vi "Kinesis-Teste-Vector-1.vi"() -> ()   [LabVIEW 2014]
doc: "André Romero - 2017\nandretec@ifsc.usp.br"
uses:
  C:/users-lab/Andre/GITs/andretec/Thorlabs-Vector-Move/kinesisTec/Kinesis/Thorlabs.MotionControl.Controls.dll
  Kinesis/Thorlabs.MotionControl.Controls.dll
  C:/users-lab/Andre/GITs/andretec/Thorlabs-Vector-Move/kinesisTec/Kinesis/Thorlabs.MotionControl.TCube.DCServoCLI.dll
  Kinesis/Thorlabs.MotionControl.TCube.DCServoCLI.dll
  C:/users-lab/Andre/GITs/andretec/Thorlabs-Vector-Move/kinesisTec/Kinesis/Thorlabs.MotionControl.GenericMotorCLI.dll
  Kinesis/Thorlabs.MotionControl.GenericMotorCLI.dll
  Basic-VIs/motorsGlobalVar.vi
  <vilib>/Instr/_visa.llb/VISA Configure Serial Port (Instr).vi
panel:
  out "IsAtHWLimit":bool
  out "CanMoveContinuous":bool
  out "GetLimitsSoftwareApproachPolicy":i16(ring) items=["DisallowIllegalMoves", "AllowPartialMoves", "AllowAllMoves"]
  in  "stop":bool
  in  "Adjust Motors":bool
  out "Process time":string="0:00:50"
  out "Progress %":dbl(slide) scale=0.0..100.0
  out "XY Graph":cluster{"Graph X":dbl[], "Graph Y":dbl[]}(graph)
  in  "Swap XY":bool
  out "stop cronometro":bool=TRUE
  in  "Stop Button":bool
  in  "Graph Y":dbl[](array[numeric])=[0.0, 0.0, 6.6674440298507465, 6.6674440298507465, 6.6674440298507465, 6.6674440298507465, 6.6674440298507465, 6.6674440298507465, 6.6674440298507465, 6.6674440298507465, 6.6674440298507465, 6.6674440298507465, 6.6674440298507465, 6.6674440298507465, 6.6674440298507465, 6.6674440298507465, 6.6674440298507465, 6.6674440298507465, 6.6674440298507465, 6.6674440298507465, 6.6674440298507465, 6.6674440298507465, 6.6674440298507465, 6.6674440298507465, 6.6674440298507465, 6.6674440298507465, 6.6674440298507465, 6.6674440298507465, 6.6674440298507465, 6.6674440298507465, 6.6674440298507465, 6.6674440298507465, 6.6674440298507465, 6.6674440298507465, 6.6674440298507465, 6.6674440298507465, 6.6674440298507465, 6.6674440298507465, 6.6674440298507465, 6.6674440298507465, 6.6674440298507465, 6.6674440298507465, 6.6674440298507465, 6.673128498134329, 6.673128498134329, 6.673128498134329, 6.673128498134329, 6.673128498134329, 6.687354244402985, 6.687354244402985, 6.687354244402985, 6.687354244402985, 6.687354244402985, 6.692543143656716, 6.692543143656716, 6.692543143656716, 6.692543143656716, 6.692543143656716, 6.692543143656716, 6.692543143656716, 6.692543143656716, 6.692543143656716, 6.692543143656716, 6.692543143656716, 6.692543143656716, 6.691522854477612, 6.691522854477612, 6.691522854477612, 6.691522854477612, 6.691522854477612, 6.680183069029851, 6.680183069029851, 6.680183069029851, 6.680183069029851, 6.680183069029851, 6.658640391791045, 6.658640391791045, 6.658640391791045, 6.658640391791045, 6.658640391791045, 6.644793610074627, 6.644793610074627, 6.644793610074627, 6.644793610074627, 6.644793610074627, 6.642490671641791, 6.642490671641791, 6.642490671641791, 6.642490671641791, 6.642490671641791, 6.642490671641791, 6.642490671641791, 6.642490671641791, 6.642490671641791, 6.642490671641791, 6.642490671641791, 6.642490671641791, 6.642490671641791, 6.642490671641791, 6.642490671641791, 6.647825326492537, 6.647825326492537, 6.647825326492537, 6.647825326492537, 6.647825326492537, 6.66543260261194, 6.66543260261194, 6.66543260261194, 6.66543260261194, 6.66543260261194, 6.685226212686567, 6.685226212686567, 6.685226212686567, 6.685226212686567, 6.685226212686567, 6.692484841417911, 6.692484841417911, 6.692484841417911, 6.692484841417911, 6.692484841417911, 6.692543143656716, 6.692543143656716, 6.692543143656716, 6.692543143656716, 6.692543143656716, 6.692543143656716, 6.692543143656716, 6.691464552238806, 6.691464552238806, 6.691464552238806, 6.691464552238806, 6.691464552238806, 6.679833255597015, 6.679833255597015, 6.679833255597015, 6.679833255597015, 6.679833255597015, 6.658057369402985, 6.658057369402985, 6.658057369402985, 6.658057369402985, 6.658057369402985, 6.644647854477612, 6.644647854477612, 6.644647854477612, 6.644647854477612, 6.644647854477612, 6.642548973880597, 6.642548973880597, 6.642548973880597, 6.642548973880597, 6.642548973880597, 6.642519822761194, 6.642519822761194, 6.642519822761194, 6.642519822761194, 6.642519822761194, 6.642519822761194, 6.642519822761194, 6.642519822761194, 6.643569263059701, 6.643569263059701, 6.643569263059701, 6.643569263059701, 6.643569263059701, 6.655521222014926, 6.655521222014926, 6.655521222014926, 6.655521222014926, 6.655521222014926, 6.677180503731344, 6.677180503731344, 6.677180503731344, 6.677180503731344, 6.677180503731344, 6.690531716417911, 6.690531716417911, 6.690531716417911, 6.690531716417911, 6.690531716417911, 6.692572294776119, 6.692572294776119, 6.692572294776119, 6.692572294776119, 6.692572294776119, 6.692572294776119, 6.692572294776119, 6.692572294776119, 6.692572294776119, 6.692572294776119, 6.692572294776119, 6.692572294776119, 6.691522854477612, 6.691522854477612, 6.691522854477612, 6.691522854477612, 6.691522854477612, 6.680008162313433, 6.680008162313433, 6.680008162313433, 6.680008162313433, 6.680008162313433, 6.668668376865671, 6.668668376865671, 6.668668376865671, 6.668668376865671, 6.668668376865671, 6.667502332089552, 6.667502332089552, 6.667502332089552, 6.667502332089552, 6.667502332089552, 6.667502332089552, 6.667502332089552, 6.667502332089552, 6.667502332089552, 6.667502332089552, 6.667502332089552, 6.667502332089552, 6.667531483208955, 6.667531483208955, 6.667531483208955, 6.667531483208955, 6.667531483208955, 6.667531483208955, 6.667531483208955, 6.667531483208955, 6.667531483208955, 6.667531483208955, 6.667531483208955, 6.667531483208955, 6.667531483208955, 6.667531483208955, 6.667531483208955, 6.667531483208955, 6.667531483208955, 6.667531483208955, 6.667531483208955, 6.667531483208955, 6.667531483208955, 6.667531483208955, 6.667531483208955, 6.667531483208955, 6.667531483208955, 6.667531483208955, 6.667531483208955, 6.667531483208955, 6.667531483208955, 6.667531483208955, 6.667531483208955, 6.667531483208955, 6.667531483208955, 6.667531483208955, 6.667531483208955, 6.667531483208955, 6.667531483208955, 6.6663945895522385, 6.6663945895522385, 6.6663945895522385, 6.6663945895522385, 6.6663945895522385, 6.662051072761194, 6.662051072761194, 6.662051072761194, 6.662051072761194, 6.662051072761194, 6.644035680970149, 6.644035680970149, 6.644035680970149, 6.644035680970149, 6.644035680970149, 6.606430736940299, 6.606430736940299, 6.606430736940299, 6.606430736940299, 6.606430736940299, 6.593924906716418, 6.593924906716418, 6.593924906716418, 6.593924906716418, 6.593924906716418, 6.574539412313433, 6.574539412313433, 6.574539412313433, 6.574539412313433, 6.574539412313433, 6.567484841417911, 6.567484841417911, 6.567484841417911, 6.567484841417911, 6.567484841417911, 6.567484841417911, 6.567484841417911, 6.567484841417911, 6.567484841417911, 6.567484841417911, 6.567484841417911, 6.567513992537314, 6.567513992537314, 6.567513992537314, 6.567513992537314, 6.567513992537314, 6.567513992537314, 6.567513992537314, 6.567513992537314, 6.567513992537314, 6.567513992537314, 6.567543143656716, 6.567543143656716, 6.567543143656716, 6.567543143656716, 6.567543143656716, 6.567543143656716, 6.567543143656716, 6.567543143656716, 6.567543143656716, 6.567543143656716, 6.567543143656716, 6.567543143656716, 6.567543143656716, 6.567543143656716, 6.567543143656716, 6.567543143656716, 6.567543143656716, 6.567543143656716, 6.567543143656716, 6.567543143656716, 6.567543143656716, 6.567543143656716, 6.567543143656716, 6.567543143656716, 6.567543143656716, 6.567543143656716, 6.567543143656716, 6.567543143656716, 6.567543143656716, 6.567543143656716, 6.567543143656716, 6.567543143656716, 6.567543143656716, 6.567543143656716, 6.567543143656716, 6.567543143656716, 6.567543143656716, 6.567543143656716, 6.567543143656716, 6.567543143656716, 6.567543143656716, 6.567543143656716, 6.567543143656716, 6.567543143656716, 6.567543143656716, 6.567543143656716, 6.567543143656716, 6.567543143656716, 6.567543143656716, 6.567543143656716, 6.567543143656716, 6.567543143656716, 6.567543143656716, 6.567543143656716, 6.5667852145522385, 6.5667852145522385, 6.5667852145522385, 6.5667852145522385, 6.5667852145522385, 6.555299673507463, 6.555299673507463, 6.555299673507463, 6.555299673507463, 6.555299673507463, 6.533523787313433, 6.533523787313433, 6.533523787313433, 6.533523787313433, 6.533523787313433, 6.525186567164179, 6.525186567164179, 6.525186567164179, 6.525186567164179, 6.525186567164179, 6.517490671641791, 6.517490671641791, 6.517490671641791, 6.517490671641791, 6.517490671641791, 6.517490671641791, 6.517490671641791, 6.517490671641791, 6.517490671641791, 6.517490671641791, 6.517519822761194, 6.517519822761194, 6.517519822761194, 6.517519822761194, 6.517519822761194, 6.517519822761194, 6.517519822761194, 6.517519822761194, 6.517519822761194, 6.517519822761194, 6.517548973880597, 6.517548973880597, 6.517548973880597, 6.517548973880597, 6.517548973880597, 6.517548973880597, 6.517548973880597, 6.517548973880597, 6.517548973880597, 6.517548973880597, 6.517548973880597, 6.517548973880597, 6.517548973880597, 6.517548973880597, 6.517548973880597, 6.517548973880597, 6.517548973880597, 6.517548973880597, 6.517548973880597, 6.517548973880597, 6.517548973880597, 6.517548973880597, 6.517548973880597, 6.517548973880597, 6.517548973880597, 6.517548973880597, 6.517548973880597, 6.517548973880597, 6.517548973880597, 6.517548973880597, 6.517548973880597, 6.517548973880597, 6.517548973880597, 6.517548973880597, 6.517548973880597, 6.517548973880597, 6.517548973880597, 6.517548973880597, 6.517548973880597, 6.517548973880597, 6.517548973880597, 6.517548973880597, 6.517548973880597, 6.517548973880597, 6.517548973880597, 6.517548973880597, 6.517548973880597, 6.517548973880597, 6.517548973880597, 6.517548973880597, 6.517548973880597, 6.517548973880597, 6.517548973880597, 6.517548973880597, 6.517548973880597, 6.517548973880597, 6.517548973880597, 6.517548973880597, 6.517548973880597, 6.517548973880597, 6.516674440298507, 6.516674440298507, 6.516674440298507, 6.516674440298507, 6.516674440298507, 6.504897388059701, 6.504897388059701, 6.504897388059701, 6.504897388059701, 6.504897388059701, 6.481926305970149, 6.481926305970149, 6.481926305970149, 6.481926305970149, 6.481926305970149, 6.456943796641791, 6.456943796641791, 6.456943796641791, 6.456943796641791, 6.456943796641791, 6.4330690298507465, 6.4330690298507465, 6.4330690298507465, 6.4330690298507465, 6.4330690298507465, 6.419717817164179, 6.419717817164179, 6.419717817164179, 6.419717817164179, 6.419717817164179, 6.417473180970149, 6.417473180970149, 6.417473180970149, 6.417473180970149, 6.417473180970149, 6.417473180970149]
  in  "Graph X":dbl[](array[numeric])=[0.0, 0.0, 3.605935167910448, 3.605935167910448, 3.605935167910448, 3.605935167910448, 3.605935167910448, 3.609987173507463, 3.609987173507463, 3.609987173507463, 3.609987173507463, 3.609987173507463, 3.627157182835821, 3.627157182835821, 3.627157182835821, 3.627157182835821, 3.627157182835821, 3.6520813899253732, 3.6520813899253732, 3.6520813899253732, 3.6520813899253732, 3.6520813899253732, 3.6770930503731343, 3.6770930503731343, 3.6770930503731343, 3.6770930503731343, 3.6770930503731343, 3.697323927238806, 3.697323927238806, 3.697323927238806, 3.697323927238806, 3.697323927238806, 3.705311333955224, 3.705311333955224, 3.705311333955224, 3.705311333955224, 3.705311333955224, 3.705311333955224, 3.705311333955224, 3.705311333955224, 3.705311333955224, 3.705311333955224, 3.705311333955224, 3.7063024720149254, 3.7063024720149254, 3.7063024720149254, 3.7063024720149254, 3.7063024720149254, 3.7175839552238807, 3.7175839552238807, 3.7175839552238807, 3.7175839552238807, 3.7175839552238807, 3.7291861007462686, 3.7291861007462686, 3.7291861007462686, 3.7291861007462686, 3.7291861007462686, 3.7303521455223883, 3.7303521455223883, 3.7303521455223883, 3.7303521455223883, 3.7303521455223883, 3.7303521455223883, 3.7303521455223883, 3.7303521455223883, 3.7303521455223883, 3.7303521455223883, 3.7303521455223883, 3.7303521455223883, 3.7366779384328357, 3.7366779384328357, 3.7366779384328357, 3.7366779384328357, 3.7366779384328357, 3.7554221082089554, 3.7554221082089554, 3.7554221082089554, 3.7554221082089554, 3.7554221082089554, 3.774137126865672, 3.774137126865672, 3.774137126865672, 3.774137126865672, 3.774137126865672, 3.7803463152985075, 3.7803463152985075, 3.7803463152985075, 3.7803463152985075, 3.7803463152985075, 3.7803463152985075, 3.7803463152985075, 3.7803463152985075, 3.7803463152985075, 3.7803463152985075, 3.7803463152985075, 3.7803463152985075, 3.7803463152985075, 3.7803463152985075, 3.7803463152985075, 3.781803871268657, 3.781803871268657, 3.781803871268657, 3.781803871268657, 3.781803871268657, 3.7941930970149254, 3.7941930970149254, 3.7941930970149254, 3.7941930970149254, 3.7941930970149254, 3.816027285447761, 3.816027285447761, 3.816027285447761, 3.816027285447761, 3.816027285447761, 3.828678871268657, 3.828678871268657, 3.828678871268657, 3.828678871268657, 3.828678871268657, 3.8303404850746268, 3.8303404850746268, 3.8303404850746268, 3.8303404850746268, 3.8303404850746268, 3.8303404850746268, 3.8303404850746268, 3.8303404850746268, 3.8303404850746268, 3.8303404850746268, 3.8303404850746268, 3.8303404850746268, 3.8368703358208953, 3.8368703358208953, 3.8368703358208953, 3.8368703358208953, 3.8368703358208953, 3.8447994402985075, 3.8447994402985075, 3.8447994402985075, 3.8447994402985075, 3.8447994402985075, 3.866633628731343, 3.866633628731343, 3.866633628731343, 3.866633628731343, 3.866633628731343, 3.8803346548507465, 3.8803346548507465, 3.8803346548507465, 3.8803346548507465, 3.8803346548507465, 3.8803346548507465, 3.8803346548507465, 3.8803346548507465, 3.8803346548507465, 3.8803346548507465, 3.8803346548507465, 3.8803346548507465, 3.8803346548507465, 3.8803346548507465, 3.8803346548507465, 3.8803346548507465, 3.8803346548507465, 3.8803346548507465, 3.886631296641791, 3.886631296641791, 3.886631296641791, 3.886631296641791, 3.886631296641791, 3.9054046175373136, 3.9054046175373136, 3.9054046175373136, 3.9054046175373136, 3.9054046175373136, 3.92411963619403, 3.92411963619403, 3.92411963619403, 3.92411963619403, 3.92411963619403, 3.9303288246268657, 3.9303288246268657, 3.9303288246268657, 3.9303288246268657, 3.9303288246268657, 3.9303288246268657, 3.9303288246268657, 3.9303288246268657, 3.9303288246268657, 3.9303288246268657, 3.9303288246268657, 3.9303288246268657, 3.9303288246268657, 3.9303288246268657, 3.9303288246268657, 3.9303288246268657, 3.9303288246268657, 3.936800373134328, 3.936800373134328, 3.936800373134328, 3.936800373134328, 3.936800373134328, 3.9445545708955225, 3.9445545708955225, 3.9445545708955225, 3.9445545708955225, 3.9445545708955225, 3.95536963619403, 3.95536963619403, 3.95536963619403, 3.95536963619403, 3.95536963619403, 3.95536963619403, 3.95536963619403, 3.95536963619403, 3.95536963619403, 3.95536963619403, 3.95536963619403, 3.95536963619403, 3.956652285447761, 3.956652285447761, 3.956652285447761, 3.956652285447761, 3.956652285447761, 3.961141557835821, 3.961141557835821, 3.961141557835821, 3.961141557835821, 3.961141557835821, 3.9795067630597014, 3.9795067630597014, 3.9795067630597014, 3.9795067630597014, 3.9795067630597014, 4.004518423507463, 4.004518423507463, 4.004518423507463, 4.004518423507463, 4.004518423507463, 4.0406366604477615, 4.0406366604477615, 4.0406366604477615, 4.0406366604477615, 4.0406366604477615, 4.048624067164179, 4.048624067164179, 4.048624067164179, 4.048624067164179, 4.048624067164179, 4.0553579757462686, 4.0553579757462686, 4.0553579757462686, 4.0553579757462686, 4.0553579757462686, 4.0553579757462686, 4.0553579757462686, 4.055387126865671, 4.055387126865671, 4.055387126865671, 4.055387126865671, 4.055387126865671, 4.055387126865671, 4.055387126865671, 4.055387126865671, 4.055387126865671, 4.055387126865671, 4.0553579757462686, 4.0553579757462686, 4.0553579757462686, 4.0553579757462686, 4.0553579757462686, 4.0553579757462686, 4.0553579757462686, 4.0553579757462686, 4.0553579757462686, 4.0553579757462686, 4.0553579757462686, 4.0553579757462686, 4.0553579757462686, 4.0553579757462686, 4.0553579757462686, 4.0553579757462686, 4.0553579757462686, 4.0553579757462686, 4.0553579757462686, 4.0553579757462686, 4.0553579757462686, 4.0553579757462686, 4.0553579757462686, 4.0553579757462686, 4.0553579757462686, 4.0553579757462686, 4.0553579757462686, 4.0553579757462686, 4.0553579757462686, 4.0553579757462686, 4.0553579757462686, 4.061800373134329, 4.061800373134329, 4.061800373134329, 4.061800373134329, 4.061800373134329, 4.06972947761194, 4.06972947761194, 4.06972947761194, 4.06972947761194, 4.06972947761194, 4.091534514925373, 4.091534514925373, 4.091534514925373, 4.091534514925373, 4.091534514925373, 4.105352145522388, 4.105352145522388, 4.105352145522388, 4.105352145522388, 4.105352145522388, 4.105381296641791, 4.105381296641791, 4.105381296641791, 4.105381296641791, 4.105381296641791, 4.105381296641791, 4.105381296641791, 4.1050897854477615, 4.1050897854477615, 4.1050897854477615, 4.1050897854477615, 4.1050897854477615, 4.0951784048507465, 4.0951784048507465, 4.0951784048507465, 4.0951784048507465, 4.0951784048507465, 4.073489972014926, 4.073489972014926, 4.073489972014926, 4.073489972014926, 4.073489972014926, 4.060954990671642, 4.060954990671642, 4.060954990671642, 4.060954990671642, 4.060954990671642, 4.023874766791045, 4.023874766791045, 4.023874766791045, 4.023874766791045, 4.023874766791045, 4.008687033582089, 4.008687033582089, 4.008687033582089, 4.008687033582089, 4.008687033582089, 4.005363805970149, 4.005363805970149, 4.005363805970149, 4.005363805970149, 4.005363805970149, 4.005363805970149, 4.005363805970149, 4.005363805970149, 4.005363805970149, 4.005363805970149, 4.005363805970149, 4.005363805970149, 4.005363805970149, 4.005363805970149, 4.005363805970149, 4.005363805970149, 4.005363805970149, 4.005392957089552, 4.005392957089552, 4.005392957089552, 4.005392957089552, 4.005392957089552, 4.005392957089552, 4.005392957089552, 4.005392957089552, 4.005392957089552, 4.005392957089552, 4.005392957089552, 4.005392957089552, 4.005392957089552, 4.005392957089552, 4.005392957089552, 4.005392957089552, 4.005392957089552, 4.005392957089552, 4.005392957089552, 4.005392957089552, 4.011631296641791, 4.011631296641791, 4.011631296641791, 4.011631296641791, 4.011631296641791, 4.019472947761194, 4.019472947761194, 4.019472947761194, 4.019472947761194, 4.019472947761194, 4.042852145522388, 4.042852145522388, 4.042852145522388, 4.042852145522388, 4.042852145522388, 4.080398787313433, 4.080398787313433, 4.080398787313433, 4.080398787313433, 4.080398787313433, 4.099113805970149, 4.099113805970149, 4.099113805970149, 4.099113805970149, 4.099113805970149, 4.103777985074627, 4.103777985074627, 4.103777985074627, 4.103777985074627, 4.103777985074627, 4.105410447761194, 4.105410447761194, 4.105410447761194, 4.105410447761194, 4.105410447761194, 4.105410447761194, 4.105410447761194, 4.105410447761194, 4.105381296641791, 4.105381296641791, 4.105381296641791, 4.105381296641791, 4.105381296641791, 4.098297574626866, 4.098297574626866, 4.098297574626866, 4.098297574626866, 4.098297574626866, 4.089989505597015, 4.089989505597015, 4.089989505597015, 4.089989505597015, 4.089989505597015, 4.06083838619403, 4.06083838619403, 4.06083838619403, 4.06083838619403, 4.06083838619403, 4.0553579757462686, 4.0553579757462686, 4.0553579757462686, 4.0553579757462686, 4.0553579757462686, 4.0553579757462686, 4.0553579757462686, 4.0553579757462686, 4.0553579757462686, 4.0553579757462686, 4.0553579757462686, 4.0553579757462686, 4.055387126865671, 4.055387126865671, 4.055387126865671, 4.055387126865671, 4.055387126865671, 4.055416277985074, 4.055416277985074, 4.055416277985074, 4.055416277985074, 4.055416277985074, 4.055416277985074, 4.055416277985074, 4.055416277985074, 4.055416277985074, 4.055416277985074, 4.055416277985074, 4.055416277985074, 4.055416277985074, 4.055416277985074, 4.055416277985074, 4.055416277985074, 4.055416277985074, 4.055416277985074, 4.055416277985074, 4.055416277985074, 4.055416277985074, 4.055416277985074, 4.055416277985074, 4.055416277985074, 4.055416277985074, 4.055416277985074, 4.055416277985074, 4.055416277985074, 4.055416277985074, 4.055416277985074, 4.055416277985074]
  out "GetPOS Y":dbl=6.417473180970149 format="%_6f"
  out "GetPOS X":dbl=4.055416277985074 format="%#_6f"
  out ".NET Refnum out 2":refnum<k24>
  out ".NET Refnum out 1":refnum<k24>
  out "Motor 2":bool
  out "Motor 1":bool
  in  "Acceleration (mm/s)":dbl=0.05
  in  "Iniciar":bool
  in  "Velocity (mm/s)":sgl=0.05
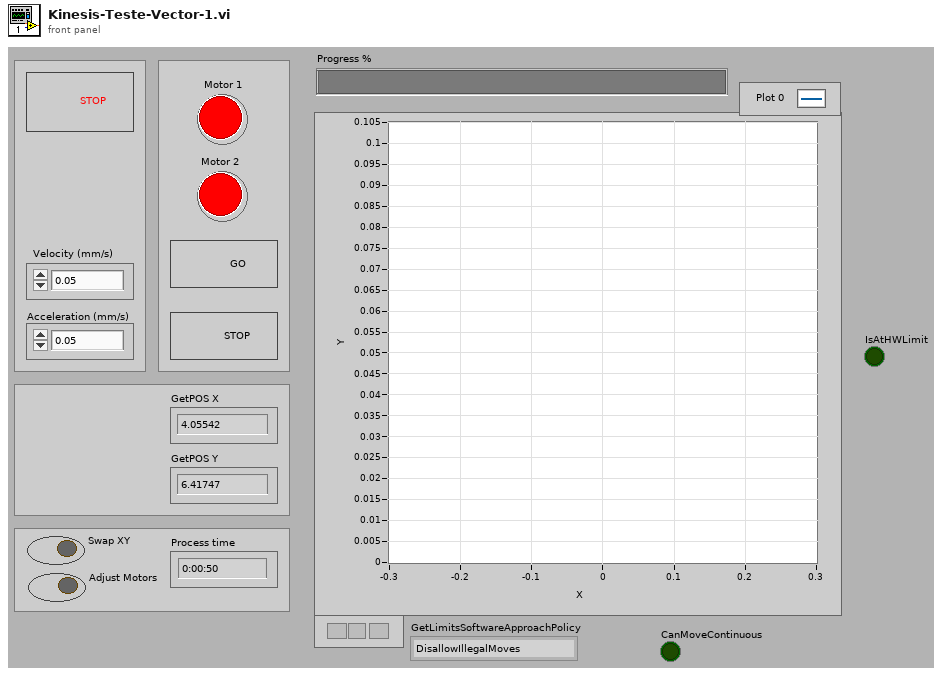
[diagram p1: front panel]
types:
  T1 = enum8{"Enabled", "Disabled", "Disabled and Grayed Out"}
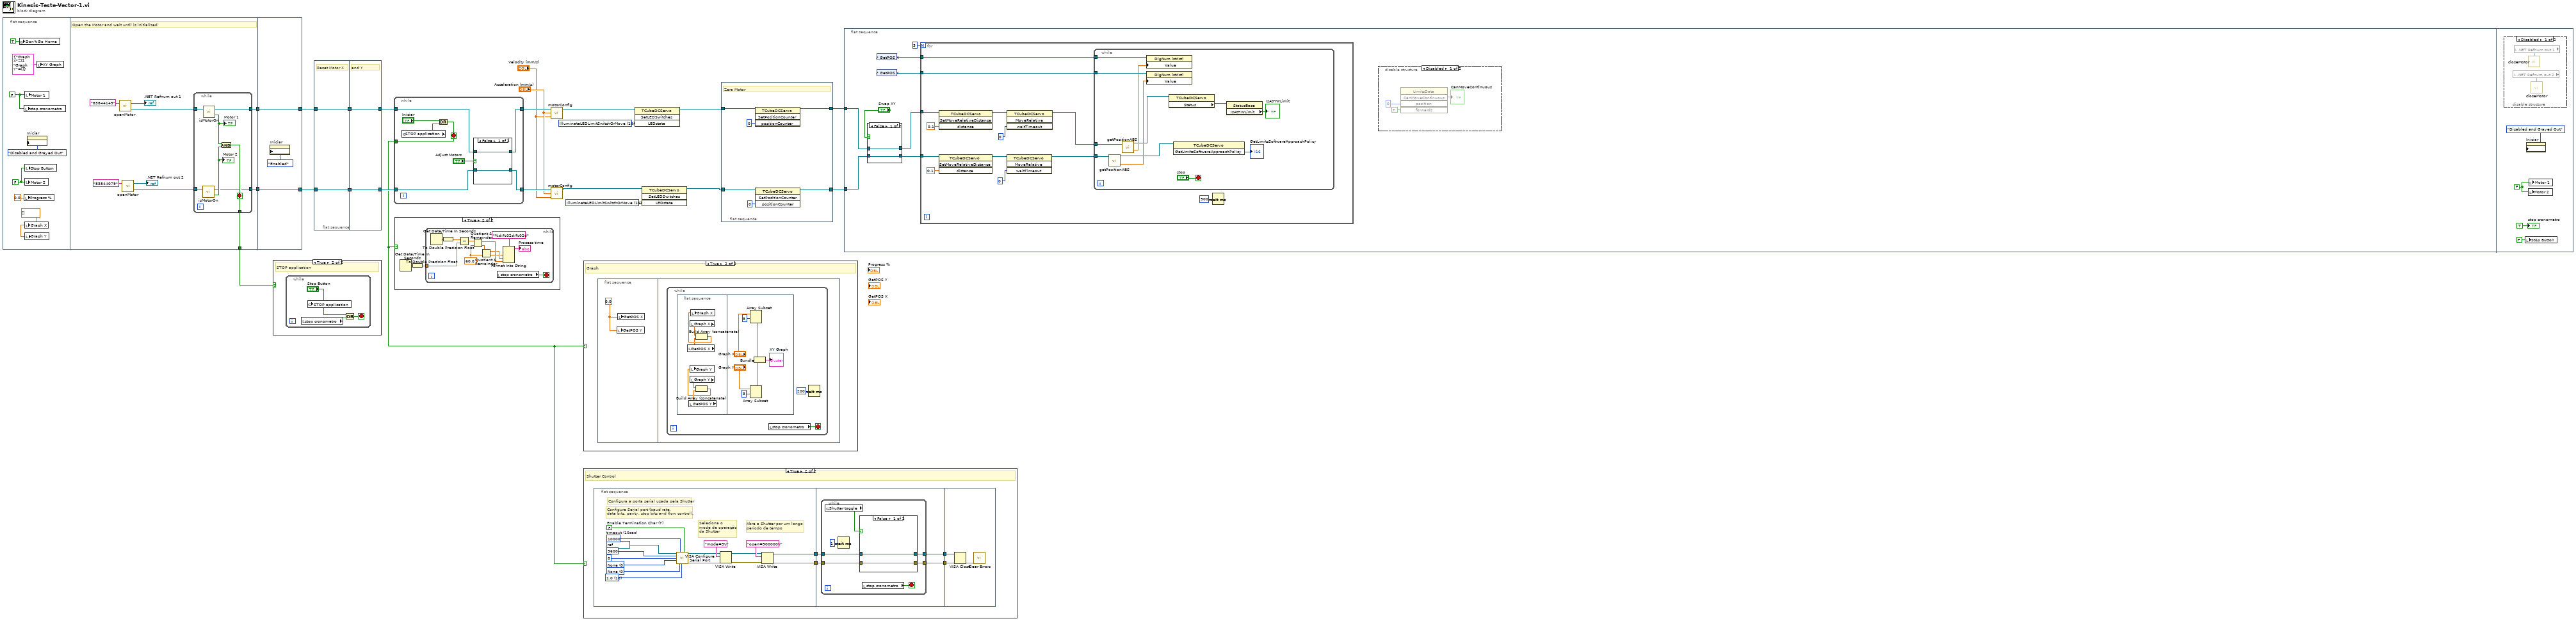
[diagram p0: block diagram]
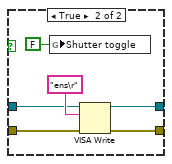
[diagram p3: hidden frame]
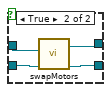
[diagram p7: hidden frame]
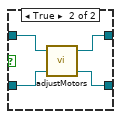
[diagram p10: hidden frame]
diagram:
  w3 = 10 items=["None"=0, "FlashLEDIdent"=1, "IlluminateLEDLimitSwitch"=2, "IlluminateLEDIdentOrLimitSwitch"=3, "IlluminateLEDMove"=8, "IlluminateLEDIdentOrMove"=9, "IlluminateLEDLimitSwitchOrMove"=10, "IlluminateLEDAny"=11] ("LEDstate")
  w4 = 10 items=["None"=0, "FlashLEDIdent"=1, "IlluminateLEDLimitSwitch"=2, "IlluminateLEDIdentOrLimitSwitch"=3, "IlluminateLEDMove"=8, "IlluminateLEDIdentOrMove"=9, "IlluminateLEDLimitSwitchOrMove"=10, "IlluminateLEDAny"=11] ("LEDstate")
  n1 = flat-sequence {
    tunnel: [w38] -> w12
    tunnel: [w37] -> w11
    tunnel: [w36] -> w10
    tunnel: [w47] -> w15
    tunnel: [w48] -> w16
    tunnel: w12 -> [w48]
    tunnel: w11 -> [w47]
    frame #0 {
      w25 = dbl[] [] ("Graph Y")
      w28 = FALSE ("Motor3\nLigado")
      w29 = FALSE
      n2 = global write "motorsGlobalVar.vi" "Don't Go Home"(TRUE ("Don't Go Home")) -> ()
      n3 = local write "stop cronometro"(w29) -> ()
      n4 = local write "Progress %"(0.0 ("Progress %")) -> ()
      n5 = local write "Motor 2"(w28) -> ()
      n6 = local write "Graph X"(w25) -> ()
      n7 = local write "Motor 1"(w29) -> ()
      n8 = local write "Stop Button"(w28) -> ()
      n9 = local write "Graph Y"(w25) -> ()
      n10 = property on="Iniciar" class="Bool (strict)"("DisabledEnum"=T1."Disabled and Grayed Out" ("Disabled")) -> ()  [unwired: 2 in, 2 out]
      n11 = local write "XY Graph"(cluster{"Graph X":dbl[], "Graph Y":dbl[]} {"Graph X"=[], "Graph Y"=[]} ("XY Graph")) -> ()
    }
    frame #1 {
      # "Open the Motor and wait until is initialized"
      n12 = call "openMotor.vi"("S/N Motor"="83844149") -> ("Device"=w34:refnum<k24>, ".NET Refnum out"=→".NET Refnum out 1":refnum<k24>)  [unwired: 1 in]
      n13 = call "openMotor.vi"("S/N Motor"="83844079") -> ("Device"=w35:refnum<k24>, ".NET Refnum out"=→".NET Refnum out 2":refnum<k24>)  [unwired: 1 in]
      n14 = while {
        tunnel: w34 -> [w43]
        tunnel: w35 -> [w42]
        tunnel: [w40] -> w38
        tunnel: [w39] -> w37
        tunnel: [w41] -> w36
        stop <- w41 stop-if-true
        n15 = call "isMotorOn.vi"("Device"=w42) -> ("isConnected"=w44:bool, "Device out"=w39:refnum<k24>)  [unwired: 1 in]
        "Motor 2" <- w44
        n16 = call "isMotorOn.vi"("Device"=w43) -> ("isConnected"=w45:bool, "Device out"=w40:refnum<k24>)  [unwired: 1 in]
        "Motor 1" <- w45
        n17 = And(x=w45, y=w44) -> (x .and. y?=w41:bool)
      }
    }
    frame #2 {
      n18 = property on="Iniciar" class="Bool (strict)"("DisabledEnum"=T1."Enabled" ("Disabled")) -> ()  [unwired: 2 in, 2 out]
    }
  }
  n19 = case shown="True" w10 {
    frame False {
    }
    frame True {
      # "STOP application"
      n20 = while {
        stop <- w50 stop-if-true
        n21 = local read "stop cronometro"() -> (w49:bool)
        n22 = global write "motorsGlobalVar.vi" "STOP application"("Stop Button") -> ()
        n23 = Or(x="Stop Button", y=w49) -> (x .or. y?=w50:bool)
      }
    }
  }
  n24 = flat-sequence {
    tunnel: w16 -> [w52]
    tunnel: w15 -> [w53]
    tunnel: [w52] -> w14
    tunnel: [w53] -> w13
    tunnel: [w55] -> w18
    tunnel: [w54] -> w17
    tunnel: w14 -> [w55]
    tunnel: w13 -> [w54]
    frame #0 {
      # "Reset Motor X"
    }
    frame #1 {
      # "and Y"
    }
  }
  n25 = while {
    tunnel: [w63] -> w9
    tunnel: w18 -> [w58]
    tunnel: w17 -> [w59]
    tunnel: [w57] -> w22
    tunnel: [w56] -> w21
    stop <- w63 stop-if-true
    n26 = global read "motorsGlobalVar.vi" "STOP application"() -> (w61:bool)
    n27 = Or(x="Iniciar", y=w61) -> (x .or. y?=w63:bool)
    n28 = case shown="False" "Adjust Motors" {
      tunnel: w59 -> [w64 w69]
      tunnel: w58 -> [w65 w68]
      tunnel: [w65 w67] -> w57
      tunnel: [w64 w66] -> w56
      frame False {
      }
      frame True {
        n29 = call "adjustMotors.vi"("Device 2"=w69, "Device 1"=w68) -> ("Device out 2"=w66:refnum<k24>, "Device out 1"=w67:refnum<k24>)  [unwired: 2 in]
      }
    }
  }
  n30 = case shown="True" w9 {
    frame False {
    }
    frame True {
      n31 = Get Date/Time In Seconds() -> (seconds since 1Jan1904=w71:timestamp)
      n32 = To Double Precision Float(number=w71) -> (double precision float=w70:dbl)
      n33 = while {
        tunnel: w70 -> [w75]
        stop <- w83 stop-if-true
        w80 = 60.0 ("y")
        n34 = Get Date/Time In Seconds() -> (seconds since 1Jan1904=w82:timestamp)
        n35 = To Double Precision Float(number=w82) -> (double precision float=w76:dbl)
        n36 = Subtract(x=w76, y=w75) -> (x-y=w74:dbl)
        n37 = Quotient & Remainder(x=w74, y=w80) -> (x-y*floor(x/y)=w79:dbl, floor(x/y)=w81:dbl)
        n38 = Quotient & Remainder(x=w81, y=w80) -> (x-y*floor(x/y)=w78:dbl, floor(x/y)=w77:dbl)
        n39 = local read "stop cronometro"() -> (w83:bool)
        n40 = Format Into String(format string="%d:%02d:%02d", w77, w78, w79) -> (resulting string=→"Process time":string)  [unwired: 2 in, 1 out]
      }
    }
  }
  n41 = call "motorConfig.vi"("Velocity"="Velocity (mm/s)", "Acceleration"="Acceleration (mm/s)", "Device in"=w22) -> ("Device out"=w6:refnum<k24>)  [unwired: 2 in]
  n42 = call "motorConfig.vi"("Velocity"="Velocity (mm/s)", "Acceleration"="Acceleration (mm/s)", "Device in"=w21) -> ("Device out"=w2:refnum<k24>)  [unwired: 2 in]
  n43 = case shown="True" w9 {
    frame False {
    }
    frame True {
      # "Graph"
      n44 = flat-sequence {
        frame #0 {
          w84 = 0.0
          n45 = local write "GetPOS Y"(w84) -> ()
          n46 = local write "GetPOS X"(w84) -> ()
        }
        frame #1 {
          n47 = while {
            stop <- w85 stop-if-true
            n48 = flat-sequence {
              frame #0 {
                n49 = local read "GetPOS X"() -> (w90:dbl)
                n50 = local read "GetPOS Y"() -> (w89:dbl)
                n51 = local read "Graph X"() -> (w92:dbl[])
                n52 = local read "Graph Y"() -> (w87:dbl[])
                n53 = Build Array (concatenate)(w92, w90) -> (w91:dbl[])
                n54 = local write "Graph X"(w91) -> ()
                n55 = Build Array (concatenate)(w87, w89) -> (w88:dbl[])
                n56 = local write "Graph Y"(w88) -> ()
              }
              frame #1 {
                n57 = Array Subset(array="Graph Y", index=3) -> (w93:dbl[])  [unwired: 1 in]
                n58 = Array Subset(array="Graph X", index=3) -> (w96:dbl[])  [unwired: 1 in]
                n59 = Bundle(w96, w93) -> (→"XY Graph":cluster{dbl[], dbl[]})  [unwired: 1 in]
              }
            }
            n60 = local read "stop cronometro"() -> (w85:bool)
            n61 = Wait (ms)(milliseconds to wait=u32 200) -> ()  [unwired: 1 out]
          }
        }
      }
    }
  }
  n62 = case shown="True" w9 {
    frame False {
    }
    frame True {
      # "Shutter Control"
      n63 = flat-sequence {
        tunnel: [w105] -> w103
        tunnel: [w104] -> w102
        tunnel: w103 -> [w123]
        tunnel: w102 -> [w120]
        tunnel: [w122] -> w101
        tunnel: [w121] -> w100
        tunnel: w101 -> [w141]
        tunnel: w100 -> [w140]
        frame #0 {
          w115 = u16 0 items=["None", "Odd", "Even", "Mark", "Space"] ("parity")
          w112 = u16 10 items=["1.0"=10, "1.5"=15, "2.0"=20] ("stop bits")
          w111 = u16 0 items=["None"=0, "XON/XOFF"=1, "RTS/CTS"=2, "DTR/DSR"=4] ("flow control")
          w113 = FALSE  # Enable Termination Char (T)
          w114 = u32 10000  # timeout (10sec)
          # "Configura a porta serial usada pela Shutter"
          # "Configure Serial port (baud rate,\ndata bits, parity, stop bits and flow control)."
          # "Seleciona o \nmode de operação\nda Shutter"
          # "Abre a Shutter por um longo\nperíodo de tempo"
          n64 = call-poly "VISA Configure Serial Port"("VISA resource name"=refnum<visa-resource-name> "COM3", "timeout (10sec)"=w114, "Enable Termination\nChar (T)"=w113, "baud rate (9600)"=u32 9600 ("baud rate"), "data bits (8)"=u16 8 ("data bits"), "parity (0:none)"=w115, "stop bits (10: 1 bit)"=w112, "flow control (0:none)"=w111) -> ("VISA resource name out"=w109:refnum<visa-resource-name>, "error out"=w108:errorcluster)  [unwired: 6 in]
          n65 = VISA Write(VISA resource name=w109, write buffer="mode=3\r", error in (no error)=w108) -> (VISA resource name out=w107:refnum<visa-resource-name>, error out=w106:errorcluster)  [unwired: 1 out]
          n66 = VISA Write(VISA resource name=w107, write buffer="open=900000\r", error in (no error)=w106) -> (VISA resource name out=w105:refnum<visa-resource-name>, error out=w104:errorcluster)  [unwired: 1 out]
        }
        frame #1 {
          n67 = while {
            tunnel: w123 -> [w130]
            tunnel: [w129] -> w122
            tunnel: [w128] -> w121
            tunnel: w120 -> [w127]
            stop <- w124 stop-if-true
            n68 = global read "motorsGlobalVar.vi" "Shutter toggle"() -> (w126:bool)
            n69 = Wait (ms)(milliseconds to wait=u32 1) -> ()  [unwired: 1 out]
            n70 = case shown="False" w126 {
              tunnel: w130 -> [w132 w137]
              tunnel: [w132 w136] -> w129
              tunnel: [w131 w135] -> w128
              tunnel: w127 -> [w131 w134]
              frame False {
              }
              frame True {
                n71 = global write "motorsGlobalVar.vi" "Shutter toggle"(FALSE ("Shutter toggle")) -> ()
                n72 = VISA Write(VISA resource name=w137, write buffer="ens\r", error in (no error)=w134) -> (VISA resource name out=w136:refnum<visa-resource-name>, error out=w135:errorcluster)  [unwired: 1 out]
              }
            }
            n73 = local read "stop cronometro"() -> (w124:bool)
          }
        }
        frame #2 {
          n74 = VISA Close(VISA resource name=w141, error in (no error)=w140) -> (error out=w139:errorcluster)
          n75 = call <vilib>:"Clear Errors.vi"("error in (no error)"=w139) -> ()  [unwired: 5 in, 2 out]
        }
      }
    }
  }
  n76 = invoke class="TCubeDCServo" method="SetLEDSwitches"(reference=w6, "LEDstate"=w4) -> (reference out=w5:refnum<k24>)  [unwired: 2 in, 3 out]
  n77 = invoke class="TCubeDCServo" method="SetLEDSwitches"(reference=w2, "LEDstate"=w3) -> (reference out=w1:refnum<k24>)  [unwired: 2 in, 3 out]
  n78 = flat-sequence {
    tunnel: w5 -> [w147]
    tunnel: w1 -> [w146]
    tunnel: [w145] -> w8
    tunnel: [w144] -> w7
    frame #0 {
      # "Zera Motor"
      n79 = invoke class="TCubeDCServo" method="SetPositionCounter"(reference=w147, "positionCounter"=0) -> (reference out=w145:refnum<k24>)  [unwired: 2 in, 3 out]
      n80 = invoke class="TCubeDCServo" method="SetPositionCounter"(reference=w146, "positionCounter"=0) -> (reference out=w144:refnum<k24>)  [unwired: 2 in, 3 out]
    }
  }
  n81 = flat-sequence {
    tunnel: w8 -> [w155]
    tunnel: w7 -> [w154]
    frame #0 {
      n82 = case shown="False" "Swap XY" {
        tunnel: w155 -> [w185 w189]
        tunnel: w154 -> [w184 w188]
        tunnel: [w185 w187] -> w150
        tunnel: [w184 w186] -> w149
        frame False {
        }
        frame True {
          n83 = call "swapMotors.vi"("Device 2"=w188, "Device 1"=w189) -> ("Device out 1"=w186:refnum<k24>, "Device out 2"=w187:refnum<k24>)  [unwired: 2 in, 2 out]
        }
      }
      n84 = control-ref of="GetPOS X"() -> (w152:refnum<vi>)
      n85 = control-ref of="GetPOS Y"() -> (w151:refnum<vi>)
      n86 = for {
        N: 3 -> [_]
        tunnel: w152 -> [w171]
        tunnel: w151 -> [w170]
        tunnel: w150 -> [w167]
        tunnel: w149 -> [w161]
        n87 = invoke class="TCubeDCServo" method="SetMoveRelativeDistance"(reference=w161, "distance"=0.1 ("position")) -> (reference out=w164:refnum<k24>)  [unwired: 2 in, 3 out]
        n88 = invoke class="TCubeDCServo" method="SetMoveRelativeDistance"(reference=w167, "distance"=0.1 ("position")) -> (reference out=w169:refnum<k24>)  [unwired: 2 in, 3 out]
        n89 = invoke class="TCubeDCServo" method="MoveRelative"(reference=w164, "waitTimeout"=0) -> (reference out=w160:refnum<k24>)  [unwired: 2 in, 3 out]
        n90 = invoke class="TCubeDCServo" method="MoveRelative"(reference=w169, "waitTimeout"=0) -> (reference out=w166:refnum<k24>)  [unwired: 2 in, 3 out]
        n91 = while {
          tunnel: w171 -> [w183]
          tunnel: w170 -> [w182]
          tunnel: w166 -> [w179]
          tunnel: w160 -> [w178]
          stop <- "stop" stop-if-true
          n92 = call "getPositionABS.vi"("Device"=w178) -> ("GetPOS"=w180:dbl, "Device out"=w174:refnum<k24>)  [unwired: 1 in]
          n93 = call "getPositionABS.vi"("Device"=w179) -> ("GetPOS"=w181:dbl, "Device out"=w176:refnum<k24>)  [unwired: 1 in]
          n94 = property class="DigNum (strict)"(reference=w183, "Value"=w181) -> ()  [unwired: 1 in, 2 out]
          n95 = property class="DigNum (strict)"(reference=w182, "Value"=w180) -> ()  [unwired: 1 in, 2 out]
          n96 = property class="TCubeDCServo"(reference=w176) -> ("Status"=w173:refnum<k24>)  [unwired: 1 in, 2 out]
          n97 = invoke class="TCubeDCServo" method="GetLimitsSoftwareApproachPolicy"(reference=w174) -> ("GetLimitsSoftwareApproachPolicy"=→"GetLimitsSoftwareApproachPolicy":i16)  [unwired: 2 in, 2 out]
          n98 = property class="StatusBase"(reference=w173) -> ("IsAtHWLimit"=→"IsAtHWLimit":bool)  [unwired: 1 in, 2 out]
        }
        n99 = Wait (ms)(milliseconds to wait=u32 500) -> ()  [unwired: 1 out]
      }
      n100 = disable-structure shown="Disabled" {
        frame Disabled {
          n101 = invoke class="LimitsData" method="CanMoveContinuous"("position"=0, "forwards"=TRUE) -> ("CanMoveContinuous"=→"CanMoveContinuous":bool)  [unwired: 3 in, 4 out]
        }
        frame Enabled {
        }
      }
    }
    frame #1 {
      w193 = FALSE
      n102 = disable-structure shown="Disabled" {
        frame Disabled {
          n103 = local read ".NET Refnum out 2"() -> (w194:refnum<k24>)
          n104 = local read ".NET Refnum out 1"() -> (w195:refnum<k24>)
          n105 = call "closeMotor.vi"(".NET Refnum in"=w195) -> ()  [unwired: 2 in]
          n106 = call "closeMotor.vi"(".NET Refnum in"=w194) -> ()  [unwired: 2 in]
        }
        frame Enabled {
        }
      }
      n107 = local write "Stop Button"(FALSE ("Stop Button")) -> ()
      n108 = property on="Iniciar" class="Bool (strict)"("DisabledEnum"=T1."Disabled and Grayed Out" ("Disabled")) -> ()  [unwired: 2 in, 2 out]
      n109 = local write "Motor 2"(w193) -> ()
      n110 = local write "Motor 1"(w193) -> ()
      "stop cronometro" <- TRUE ("stop cronometro")
    }
  }
